vi "Select next.vi"(0 "Display State In":T1={"Nspeakers"=13, "actions"=[], "Wspeaker"=13, "Wmic"=13, "sel mic"=13, "hover"={"type"=enum."None", "index"=0}, "locked"=FALSE, "states"=[], "sel speak"=13, "selected"=refnum, "Events"={"Mic change"=refnum, "Selection change"=refnum}}, 9 "Container State":T6, 11 "error in (no error)":errorcluster) -> (4 "Display State Out":T1={"Nspeakers"=13, "actions"=[], "Wspeaker"=13, "Wmic"=13, "sel mic"=13, "hover"={"type"=enum."None", "index"=0}, "locked"=FALSE, "states"=[], "sel speak"=13, "selected"=refnum, "Events"={"Mic change"=refnum, "Selection change"=refnum}}, 6 "Next":i32, 15 "error out":errorcluster)   [LabVIEW 2015, in "HRTF Config.xctl"]
uses:
  HRTF Config.xctl
  <vilib>/_xctls/Container State.ctl
  State.vi
  Hover Data.ctl
  Hover Item.ctl
  Speaker State.ctl
  Events.ctl
  Selection changed.ctl
  <vilib>/_xctls/XControlSupport.lvlib
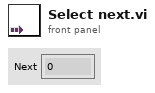
[diagram p1: front panel]
types:
  T1 = typedef "HRTF Config.xctl/State.vi" = cluster{"Nspeakers":i32, "actions":string[], "Wspeaker":i32, "Wmic":i32, "sel mic":i32, "hover":T2, "locked":bool, "states":T4[], "sel speak":i32, "selected":refnum<vi>, "Events":T5}
  T2 = typedef "HRTF Config.xctl/Hover Data.ctl" = cluster{"type":T3, "index":i32}
  T3 = typedef "HRTF Config.xctl/Hover Item.ctl" = enum16{"None", "Speaker", "Mic"}
  T4 = typedef "HRTF Config.xctl/Speaker State.ctl" = cluster{"right cal":bool, "left cal":bool, "selected":bool}
  T5 = typedef "HRTF Config.xctl/Events.ctl" = cluster{"Mic change":refnum<user-event>, "Selection change":refnum<user-event>}
  T6 = typedef "XControlSupport.lvlib/Container State.ctl" = cluster{"Indicator?":bool, "Run Mode?":bool, " Refnum":refnum<vi>}
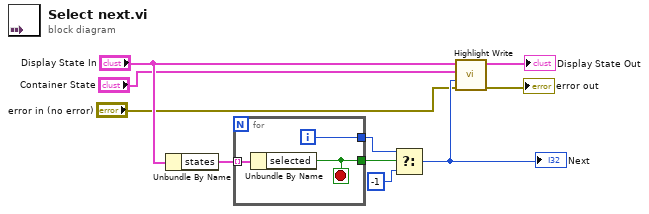
[diagram p0: block diagram]
diagram:
  n1 = Unbundle By Name("Display State In") -> ("states"=w10:T4[])
  n2 = for {
    tunnel: w10 -> [w13] mode=indexing
    tunnel: [w12] -> w8
    tunnel: [w11] -> w9
    i -> [w12]
    stop <- w11 stop-if-true
    n3 = Unbundle By Name(w13) -> ("selected"=w11:bool)
  }
  n4 = Select(t=w8, s=w9, f=-1) -> (s? t:f=w3:i32)
  "Next" <- w3
  n5 = call "Highlight Write.vi"("error in (no error)"="error in (no error)", "Value"=w3, "Container State"="Container State", "Display State In"="Display State In") -> ("error out"=→"error out":errorcluster, "Display State Out"=→"Display State Out":T1)  [unwired: 2 in]
